vi "Generate Other Event.vi"(0 "Event Number":i32) -> ()   [LabVIEW 2019]
uses:
  QCA Global.vi
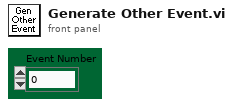
[diagram p1: front panel]
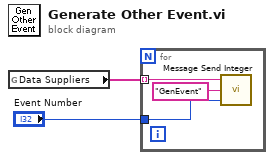
[diagram p0: block diagram]
diagram:
  n1 = global read "QCA Global.vi" "Data Suppliers"() -> (w1:string[])
  n2 = for {
    tunnel: "Event Number" -> [w4]
    tunnel: w1 -> [w3] mode=indexing
    n3 = call "Message Send Integer.vi"("Value"=w4, "Parameter"="GenEvent", "Destination"=w3) -> ()
  }
